vi "test 1.vi"(8 "error in (no error)":errorcluster caption="에러 입력(에러 없음)") -> (0 "error out":errorcluster caption="에러 출력", 1 "Home":bool)   [LabVIEW 2019]
uses:
  <vilib>/Utility/miscctls.llb/LVPointTypeDef.ctl
  RT/CANopen/State.ctl
panel:
  in  "Home Button":bool
  # "1"
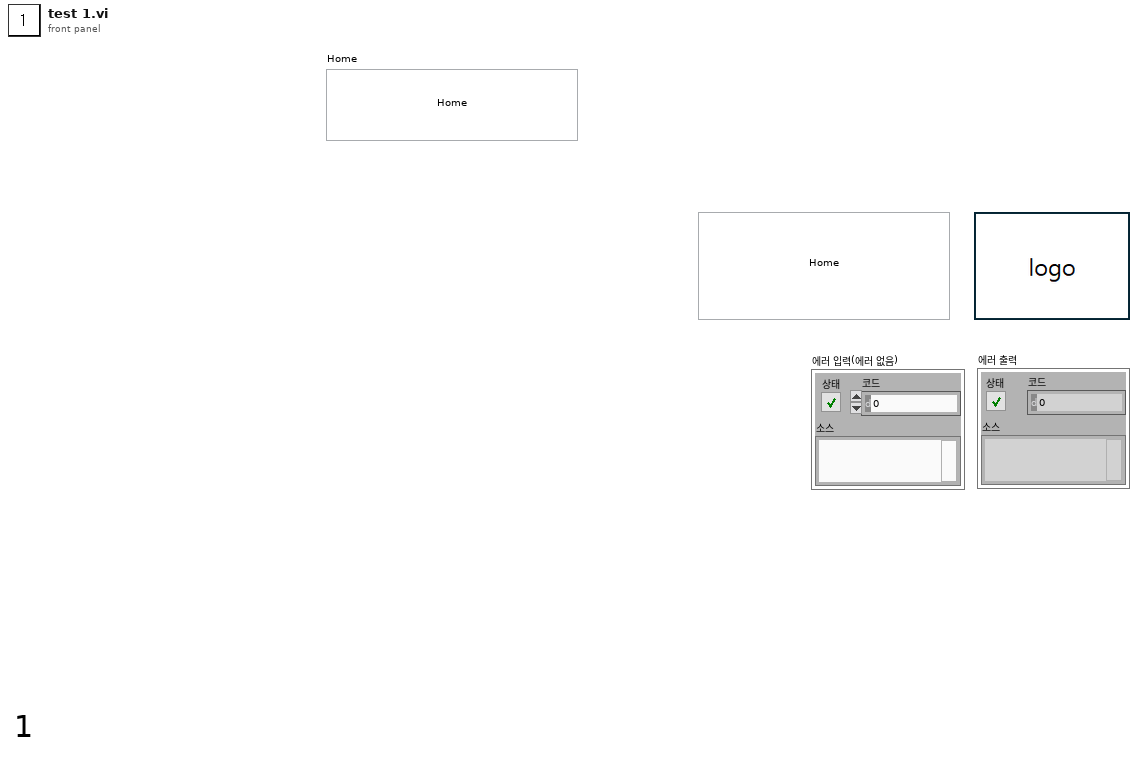
[diagram p1: front panel]
types:
  T1 = typedef "LVPointTypeDef.ctl" = cluster{"Horizontal":i16, "Vertical":i16}
  T2 = typedef "State.ctl" = enum16{"Init", "LogIn", "SignUpView", "Home", "Management_patientList", "Management_patientTrashtList", "Management_patientCreate", "Management_patientUpdate", "Management_patientTraining", "Management_patientTrainingDetail", "H-MEDI PatientList", "H-MEDI HardwareCtl", "Adjust", "FineTuning", "UserList", "UserDetail", "Exit"}
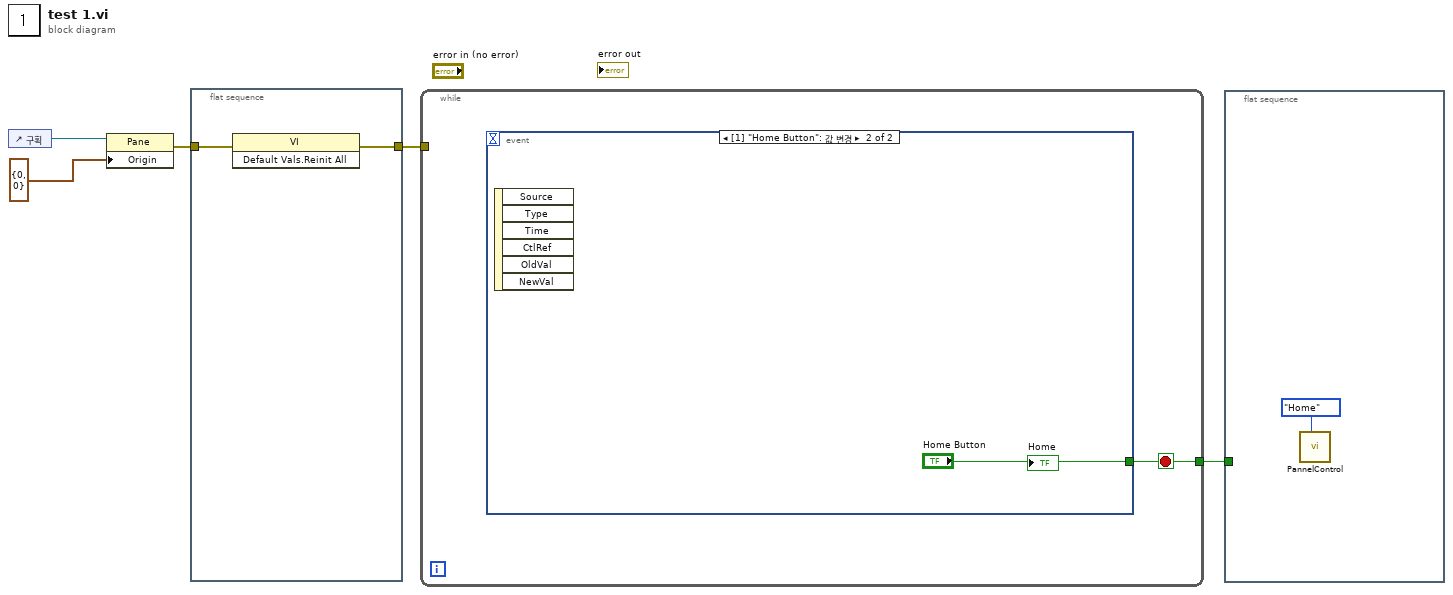
[diagram p0: block diagram]
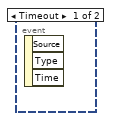
[diagram p2: hidden frame]
diagram:
  n1 = control-ref of="구획"() -> (w2:refnum<vi>)
  n2 = property class="Pane"(reference=w2, "Origin"=T1 {"Horizontal"=0, "Vertical"=0} ("원점")) -> (error out=w3:errorcluster)  [unwired: 1 in, 1 out]
  n3 = flat-sequence {
    tunnel: [w7] -> w5
    tunnel: w3 -> [w6]
    frame #0 {
      n4 = invoke class="VI" method="Default Vals.Reinit All"(error in=w6) -> (error out=w7:errorcluster)  [unwired: 2 in, 2 out]
    }
  }
  n5 = while {
    tunnel: w5 -> [_]
    tunnel: [w8] -> w1
    stop <- w8 stop-if-true
    n6 = event shown="[1] \"Home Button\": 값 변경" {
      selector: _ -> [_ _]
      dyn-events: _ -> [_ _]
      timeout: _ -> [_ _]
      tunnel: [_ "Home Button"] -> w8
      event Timeout {
        n7 = event-data() -> ()  [unwired: 1 in, 3 out]
      }
      event "Home Button": Value Change {
        n8 = event-data() -> ()  [unwired: 1 in, 6 out]
        "Home" <- "Home Button"
      }
    }
  }
  n9 = flat-sequence {
    tunnel: w1 -> [_]
    frame #0 {
      n10 = call "PannelControl.vi"("State"=State."Home") -> ()  [unwired: 10 in, 1 out]
    }
  }
